vi "Motors Position Rewrite.vi"(6 "file path":path=path "C:/LabView VIs/IPES SubVIs/saved_positions.txt", 10 "Array of Positions":string[][](array[string])) -> ()   [LabVIEW 2018]
uses:
  <vilib>/Utility/file.llb/Write To Spreadsheet File (string).vi
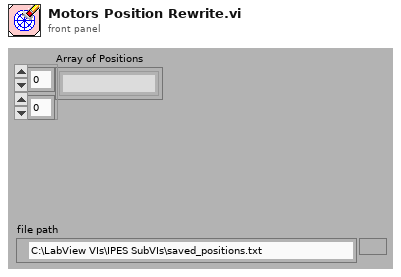
[diagram p1: front panel]
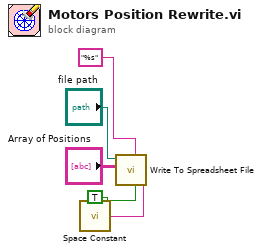
[diagram p0: block diagram]
diagram:
  n1 = call <vilib>:"Space Constant.vi"() -> ("String"=w5:string)
  n2 = call-poly <vilib>:"Write To Spreadsheet File.vi"("delimiter (\\t)"=w5, "transpose? (no:F)"=TRUE, "format (%s)"="%s" ("format (%.3f)"), "2D data"="Array of Positions", "file path (dialog if empty)"="file path") -> ()  [unwired: 3 in, 1 out]
